vi "Measure Voltage.vi"(8 "error in":errorcluster, 11 "4124 in":refnum<class "4124.lvclass">) -> (0 "error out":errorcluster, 2 "Voltage":dbl, 3 "4124 out":refnum<class "4124.lvclass">)   [LabVIEW 2018, in "4124.lvlib" / "4124.lvclass"]
uses:
  4124.lvclass
  <instrlib>/NI RMX-412x Power Supplies/NI RMX-412x Power Supplies.lvlib
  builds/Power_Supply.lvlibp/Power Supply.lvclass
  C:/Users/Ron.Dexter.LUMINARTECH/Desktop/builds/Power_Supply.lvlibp/Power Supply.lvclass
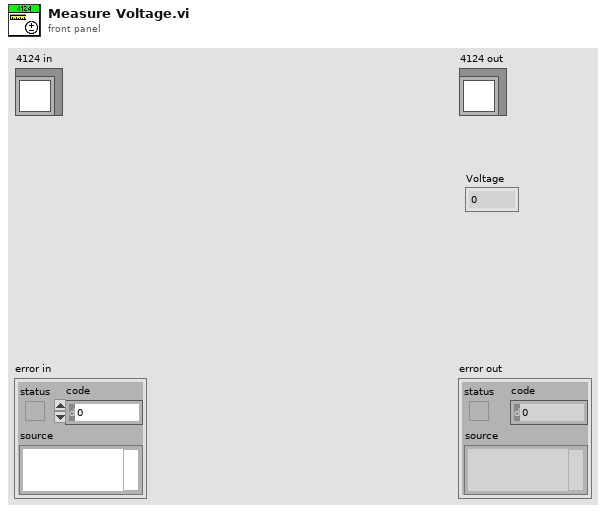
[diagram p1: front panel]
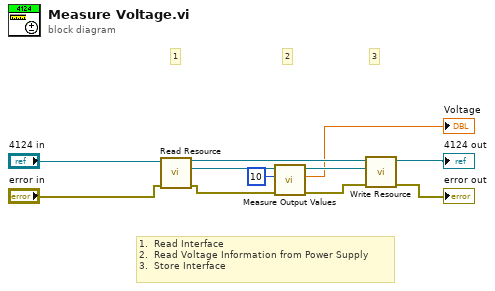
[diagram p0: block diagram]
diagram:
  # "1.  Read Interface\n2.  Read Voltage Information from Power Supply\n3.  Store Interface"
  # "3"
  # "2"
  # "1"
  n1 = call "Read Resource.vi"("error in"="error in", "Power Supply in"="4124 in") -> ("error out"=w3:errorcluster, "Resource"=w8:refnum<visa-resource-name>, "Power Supply out"=w9:refnum<class "4124.lvclass">)  [unwired: 7 in]
  n2 = call <instrlib>:"Measure Output Values.vi"("error in (no error)"=w3, "Wait Before Query (1550 ms)"=u32 10, "VISA resource name"=w8) -> ("error out"=w5:errorcluster, "Voltage Output"=→"Voltage":dbl, "VISA resource name out"=w7:refnum<visa-resource-name>)  [unwired: 5 in, 1 out]
  n3 = call "Write Resource.vi"("error in"=w5, "Resource"=w7, "Power Supply in"=w9) -> ("error out"=→"error out":errorcluster, "Power Supply out"=→"4124 out":refnum<class "4124.lvclass">)  [unwired: 7 in]
